vi "Filter Joystick Z.vi"(10 "Scale":dbl=1.0, 11 "Z In":dbl) -> (3 "Z Out":dbl)   [LabVIEW 2013]
panel:
  in  "Deadband Range":dbl=0.30000000000000004 format="%#_13g"
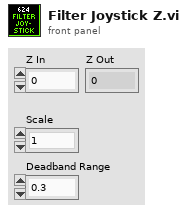
[diagram p1: front panel]
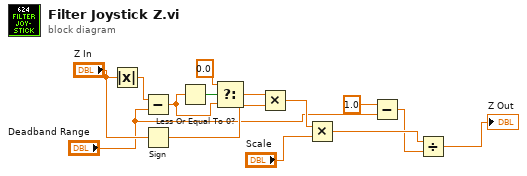
[diagram p0: block diagram]
diagram:
  n1 = Absolute Value(x="Z In") -> (abs(x)=w10:dbl)
  n2 = Subtract(x=w10, y="Deadband Range") -> (x-y=w12:dbl)
  n3 = Sign(1:"Z In") -> (0:w14:dbl)
  n4 = Less Or Equal To 0?(x=w12) -> (x <= 0?=w11:bool)
  n5 = Select(t=0.0, s=w11, f=w12) -> (s? t:f=w13:dbl)
  n6 = Multiply(x=w13, y=w14) -> (x*y=w6:dbl)
  n7 = Multiply(x=w6, y="Scale") -> (x*y=w3:dbl)
  n8 = Subtract(x=1.0, y="Deadband Range") -> (x-y=w2:dbl)
  n9 = Divide(x=w3, y=w2) -> (x/y=→"Z Out":dbl)
